vi "multiSaving.vi"() -> ()   [LabVIEW 2020]
uses:
  <vilib>/Utility/file.llb/Write Delimited Spreadsheet (DBL).vi
  <instrlib>/Ocean Optics 2000 4000/Ocean Optics 2000 4000.lvlib
panel:
  out "inner i":i32
  out "outer i":i32
  out "Spectral Waveform":cluster{dbl[], dbl[]}(graph)
  out "Array":dbl[](array[numeric])
  in  "Enable Strobe (Disabled)":bool
  in  "VISA resource name":refnum<visa-resource-name>
  out "selected path":path
  in  "inner":i32
  in  "outer":i32
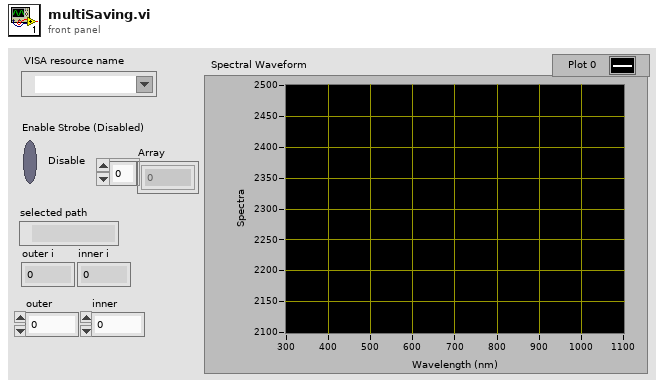
[diagram p1: front panel]
types:
  T1 = cluster{"Wavelength (nm)":dbl[], "Spectrum by Pixel Number":dbl[]}
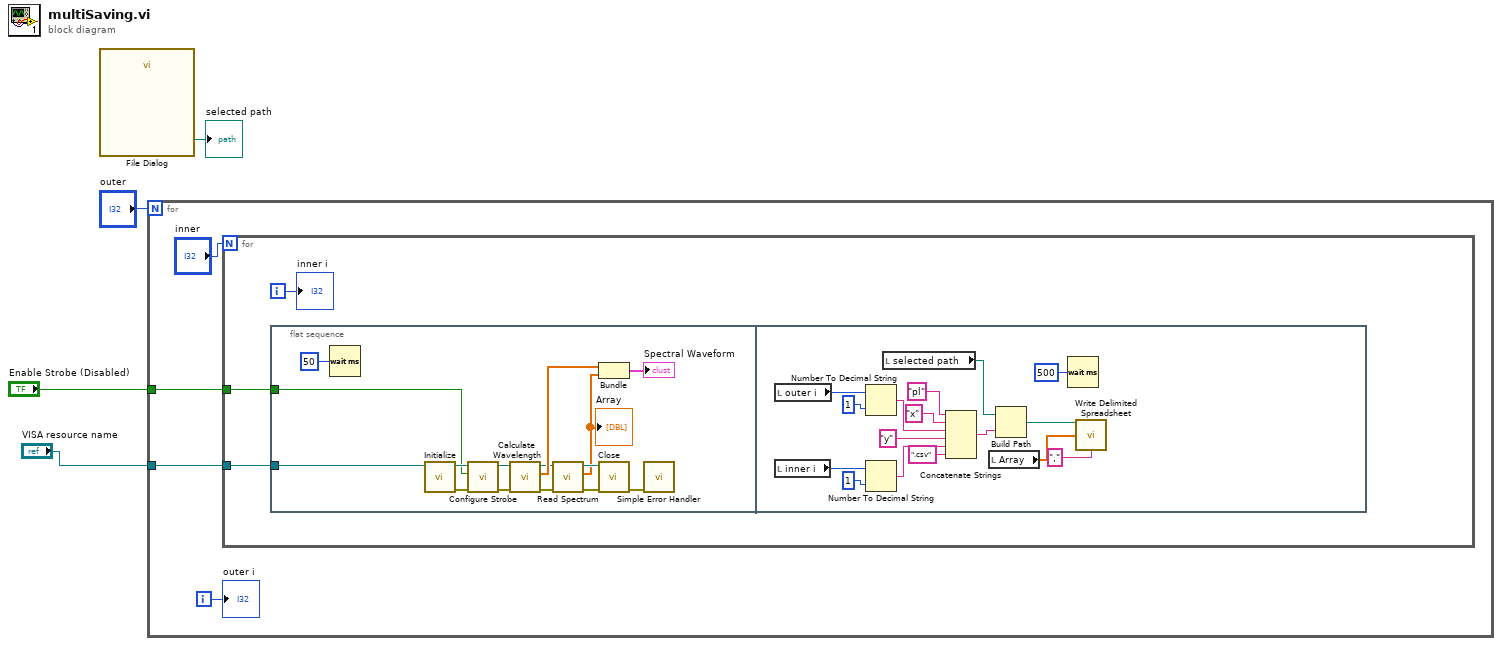
[diagram p0: block diagram]
diagram:
  n1 = call "File Dialog"() -> ("selected path"=→"selected path":path)  [unwired: 12 in, 3 out]
  n2 = for {
    N: "outer" -> [_]
    tunnel: "VISA resource name" -> [w6]
    tunnel: "Enable Strobe (Disabled)" -> [w5]
    i -> [w7]
    n3 = for {
      N: "inner" -> [_]
      tunnel: w6 -> [w10]
      tunnel: w5 -> [w9]
      i -> [w11]
      n4 = flat-sequence {
        tunnel: w10 -> [w13]
        tunnel: w9 -> [w12]
        frame #0 {
          n5 = Wait (ms)(milliseconds to wait=u32 50 ("millisecond multiple")) -> ()  [unwired: 1 out]
          n6 = call <instrlib>:"Initialize.vi"("VISA resource name"=w13) -> ("error out"=w25:errorcluster, "VISA resource name out"=w26:refnum<visa-resource-name>)  [unwired: 2 in, 7 out]
          n7 = call <instrlib>:"Configure Strobe.vi"("error in (no error)"=w25, "Enable Strobe (Disabled)"=w12, "VISA resource name"=w26) -> ("error out"=w17:errorcluster, "VISA resource name out"=w18:refnum<visa-resource-name>)  [unwired: 7 out]
          n8 = call <instrlib>:"Calculate Wavelength.vi"("error in (no error)"=w17, "VISA resource name"=w18) -> ("error out"=w19:errorcluster, "Wavelength (nm)"=w21:dbl[], "VISA resource name out"=w20:refnum<visa-resource-name>)  [unwired: 1 in, 6 out]
          n9 = call <instrlib>:"Read Spectrum.vi"("error in (no error)"=w19, "VISA resource name"=w20) -> ("error out"=w23:errorcluster, "Spectrum by Pixel Number"=w14:dbl[], "VISA resource name out"=w24:refnum<visa-resource-name>)  [unwired: 6 in, 1 out]
          "Array" <- w14
          n10 = Bundle("Wavelength (nm)"=w21, "Spectrum by Pixel Number"=w14) -> (→"Spectral Waveform":T1)  [unwired: 1 out]
          n11 = call <instrlib>:"Close.vi"("error in (no error)"=w23, "VISA resource name"=w24) -> ("error out"=w22:errorcluster)  [unwired: 9 out]
          n12 = call <vilib>:"Simple Error Handler.vi"("error in (no error)"=w22) -> ()  [unwired: 1 in, 8 out]
        }
        frame #1 {
          n13 = local read "outer i"() -> (w38:i32)
          n14 = local read "inner i"() -> (w37:i32)
          n15 = Number To Decimal String(number=w38, width (-)=i16 1) -> (decimal integer string=w34:string)
          n16 = Number To Decimal String(number=w37, width (-)=i16 1) -> (decimal integer string=w32:string)
          n17 = local read "selected path"() -> (w30:path)
          n18 = Concatenate Strings("pl", "x", w34, "y", w32, ".csv" ("string")) -> (w31:string)
          n19 = local read "Array"() -> (w41:dbl[])
          n20 = Build Path(base path=w30, name or relative path=w31) -> (appended path=w27:path)
          n21 = Wait (ms)(milliseconds to wait=u32 500) -> ()  [unwired: 1 out]
          n22 = call-poly <vilib>:"Write Delimited Spreadsheet.vi"("file path (dialog if empty)"=w27, "1D data"=w41, "delimiter (\\t)"="," ("delimiter (\\t)")) -> ()  [unwired: 11 in, 2 out]
        }
      }
      "inner i" <- w11
    }
    "outer i" <- w7
  }
